vi "ReadEmbedded.vi"(6 "timeout in ms (-1)":i32, 8 "error in (no error)":errorcluster, 11 "MAUI in":refnum<class "SMO.UI.MAUI.lvclass">) -> (0 "error out":errorcluster, 2 "Subpanels":refnum<class "SMO.UI.Embedded.lvclass">[](array[class]), 3 "MAUI out":refnum<class "SMO.UI.MAUI.lvclass">)   [LabVIEW 2019, in "SMO.UI.MAUI.lvclass"]
uses:
  SMO.UI.MAUI.lvclass
  <userlib>/LevyLab/Embedded UI/SMO.UI.Embedded/SMO.UI.Embedded.lvclass
  Typedefs/PrivateEvents--SMO.UI.MAUI.GetEmbedded.ctl
  SMO.UI.MAUI.lvclass/SMO.UI.MAUI.ctl
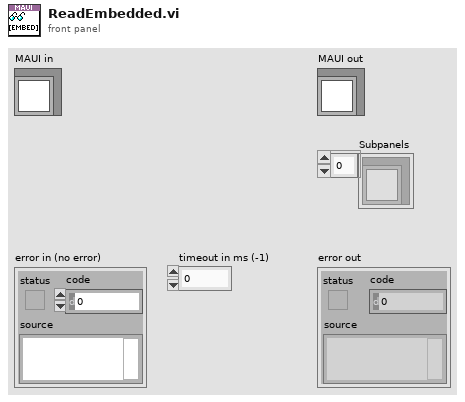
[diagram p1: front panel]
types:
  T1 = typedef "SMO.UI.MAUI.lvclass/PrivateEvents--SMO.UI.MAUI.GetEmbedded.ctl" = cluster{"notifier out":refnum<notifier>}
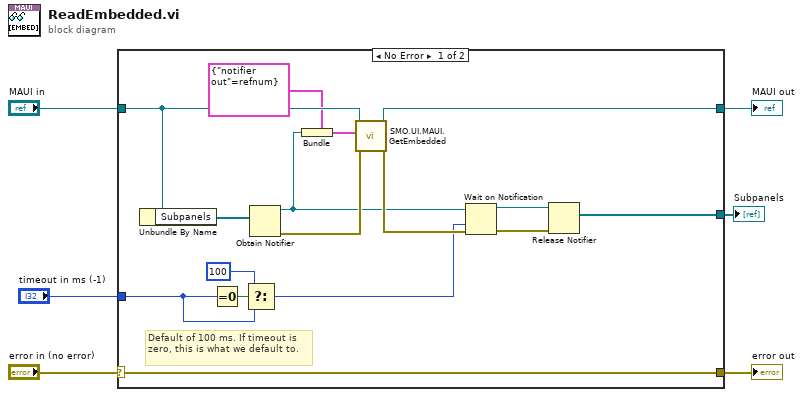
[diagram p0: block diagram]
diagram:
  n1 = case shown="No Error" "error in (no error)" {
    selector: "error in (no error)" -> [w22 w24]
    tunnel: [w22 w24] -> w6
    tunnel: [w14 w23] -> w3
    tunnel: "MAUI in" -> [w15 w23]
    tunnel: "timeout in ms (-1)" -> [w7 _]
    tunnel: [w16 _] -> w1
    frame No Error {
      # "Default of 100 ms. If timeout is zero, this is what we default to."
      n2 = Unbundle By Name(w15) -> ("Subpanels"=w18:refnum<class "SMO.UI.Embedded.lvclass">[])
      n3 = Equal To 0?(x=w7) -> (x = 0?=w8:bool)
      n4 = Select(t=100, s=w8, f=w7) -> (s? t:f=w9:i32)
      n5 = Obtain Notifier(notification data type=w18) -> (notifier out=w11:refnum<notifier>, error out=w20:errorcluster)  [unwired: 3 in, 1 out]
      n6 = Bundle(cluster=T1 {"notifier out"=refnum} ("GetEmbedded"), "notifier out"=w11) -> (w12:T1)
      n7 = call "SMO.UI.MAUI.GetEmbedded.vi"("error in (no error)"=w20, "GetEmbedded"=w12, "MAUI"=w15) -> ("error out"=w19:errorcluster, "MAUI out"=w14:refnum<class "SMO.UI.MAUI.lvclass">)  [unwired: 7 in]
      n8 = Wait on Notification(notifier=w11, timeout in ms (-1)=w9, error in (no error)=w19) -> (notifier out=w17:refnum<notifier>, error out=w21:errorcluster)  [unwired: 1 in, 2 out]
      n9 = Release Notifier(notifier=w17, error in (no error)=w21) -> (last notification=w16:refnum<class "SMO.UI.Embedded.lvclass">[])  [unwired: 1 in, 2 out]
    }
    frame Error {
    }
  }
  "error out" <- w6
  "MAUI out" <- w3
  "Subpanels" <- w1
